vi "DistToNearestSegmentEdge.vi"(9 "error in (no error)":errorcluster, 10 "UTM Location":T1 {"North" format="%#_10f"; "East" format="%#_8f"}, 11 "Obstacle.lvclass":refnum<class "Obstacle.lvclass">) -> (3 "min value":dbl)   [LabVIEW 2013, in "Obstacle.lvclass"]
doc: "Takes in Obstacle and a UTM location and returns the distance to the closest point in the object.\nPerpetrator: Michael Bocamazo"
uses:
  Obstacle.lvclass
  Data/TypeDefs/UTM Location.ctl
  Obstacle.lvclass/Obstacle.ctl
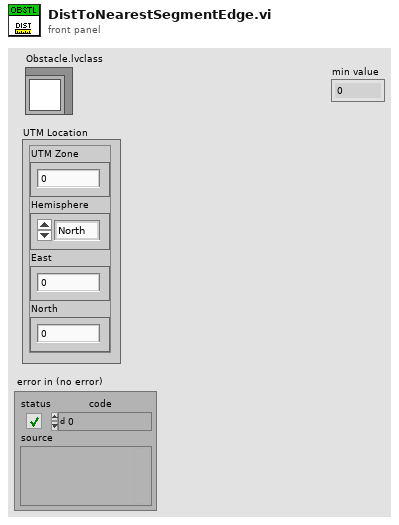
[diagram p1: front panel]
types:
  T1 = typedef "UTM Location.ctl" = cluster{"UTM Zone":dbl, "Hemisphere":enum16{"North", "South"}, "East":dbl, "North":dbl}
  T2 = cluster{"UTM Obstacle Point 2":T1, "UTM Obstacle Point 1":T1}[]
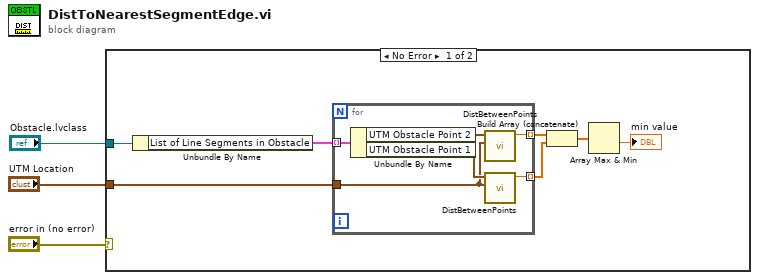
[diagram p0: block diagram]
diagram:
  n1 = case shown="No Error" "error in (no error)" {
    tunnel: "Obstacle.lvclass" -> [w10 _]
    tunnel: "UTM Location" -> [w8 _]
    frame No Error {
      n2 = Unbundle By Name(w10) -> ("List of Line Segments in Obstacle"=w9:T2)
      n3 = for {
        tunnel: w9 -> [w16] mode=indexing
        tunnel: w8 -> [w13]
        tunnel: [w12] -> w6 mode=indexing
        tunnel: [w11] -> w5 mode=indexing
        n4 = Unbundle By Name(w16) -> ("UTM Obstacle Point 2"=w15:T1, "UTM Obstacle Point 1"=w14:T1)
        n5 = call "DistBetweenPoints.vi"("UTM Location 2"=w13, "UTM Location 1"=w15) -> ("Distance from 1 to 2"=w12:dbl)  [unwired: 9 in]
        n6 = call "DistBetweenPoints.vi"("UTM Location 2"=w13, "UTM Location 1"=w14) -> ("Distance from 1 to 2"=w11:dbl)  [unwired: 9 in]
      }
      n7 = Build Array (concatenate)(w6, w5) -> (w4:dbl[])
      n8 = Array Max & Min(array=w4) -> (min value=→"min value":dbl)  [unwired: 3 out]
    }
    frame Error {
    }
  }
